vi "Read Joint Position.vi"(8 "Error In":errorcluster, 10 "Body Index":i32, 11 "JointType":T1 items=["SpineBase", "SpineMid", "Neck", "Head", "ShoulderLeft", "ElbowLeft", "WristLeft", "HandLeft", "ShoulderRight", "ElbowRight", "WristRight", "HandRight", "HipLeft", "KneeLeft", "AngleLeft", "FootLeft", "HipRight", "KneeRight", "AngleRight", "FootRight", "SpineShoulder", "HandTipLeft", "ThumbLeft", "HandTipRight", "ThumbRight"]) -> (0 "Error Out":errorcluster, 2 "Tracked?":bool, 3 "Position (Color Space)":cluster{"X":sgl, "Y":sgl})   [LabVIEW 2011, in "KinectOne.lvlib"]
doc: "Read the color space position of the specified joint."
uses:
  KinectOne.lvlib
  Private/Type Defs/JointType.ctl
panel:
  in  "Include Inferred Joints?":bool=TRUE
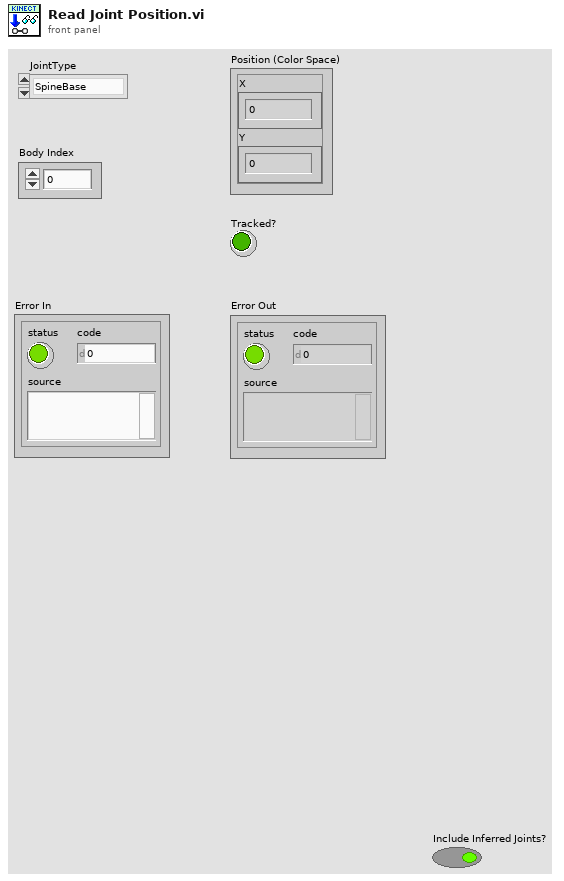
[diagram p1: front panel]
types:
  T1 = typedef "KinectOne.lvlib/JointType.ctl" = i32
  T2 = typedef "KinectOne.lvlib/Joint Position.ctl" = cluster{"Color Space Position":cluster{"X":sgl, "Y":sgl}, "Depth Space Position":cluster{"X":sgl, "Y":sgl}, "TrackingState":i32}
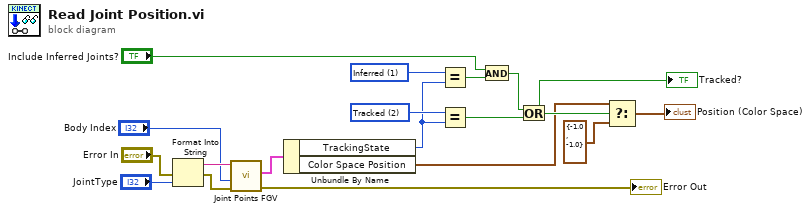
[diagram p0: block diagram]
diagram:
  w13 = 1 items=["NotTracked", "Inferred", "Tracked"] ("TrackingState")
  w14 = 2 items=["NotTracked", "Inferred", "Tracked"] ("TrackingState")
  n1 = Format Into String(error in="Error In", "JointType") -> (resulting string=w16:string, error out=w17:errorcluster)  [unwired: 2 in]
  n2 = call "Joint Points FGV.vi"("error in (no error)"=w17, "Body Index"="Body Index", "name"=w16) -> ("error out"=→"Error Out":errorcluster, "Joint Position"=w18:T2)  [unwired: 7 in]
  n3 = Unbundle By Name(w18) -> ("TrackingState"=w8:i32, "Color Space Position"=w5:cluster{"X":sgl, "Y":sgl})
  n4 = Equal?(x=w13, y=w8) -> (x = y?=w12:bool)
  n5 = Equal?(x=w14, y=w8) -> (x = y?=w9:bool)
  n6 = And(x="Include Inferred Joints?", y=w12) -> (x .and. y?=w10:bool)
  n7 = Or(x=w10, y=w9) -> (x .or. y?=w6:bool)
  "Tracked?" <- w6
  n8 = Select(t=w5, s=w6, f=cluster{"X":sgl, "Y":sgl} {"X"=-1.0, "Y"=-1.0}) -> (s? t:f=→"Position (Color Space)":cluster{"X":sgl, "Y":sgl})
